vi "AlazarFFTSetScalingAndSlicing.vi"(2 "error in (no error)":errorcluster, 3 "loge_ampl_mult":sgl, 4 "slice_pos":u8, 5 "DSP Handle":u64) -> (0 "error out":errorcluster, 1 "DSP Handle":u64)   [LabVIEW 2018]
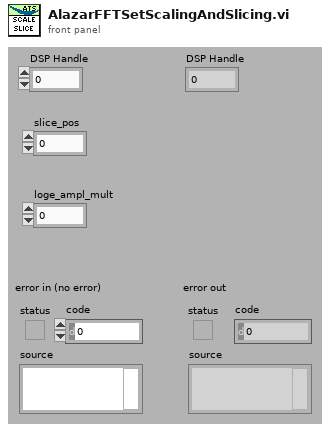
[diagram p1: front panel]
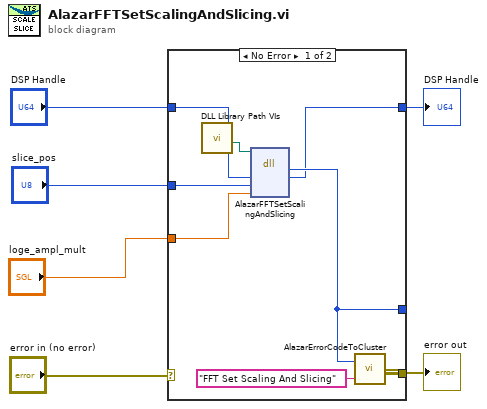
[diagram p0: block diagram]
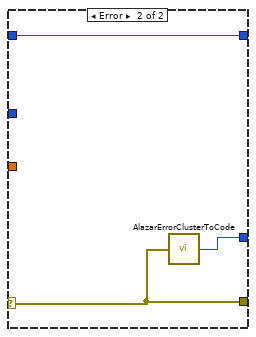
[diagram p2: hidden frame]
diagram:
  n1 = case shown="No Error" "error in (no error)" {
    selector: "error in (no error)" -> [_ w17]
    tunnel: [w11 w17] -> w5
    tunnel: [w13 w16] -> _
    tunnel: "DSP Handle" -> [w14 w15]
    tunnel: [w10 w15] -> w3
    tunnel: "slice_pos" -> [w9 _]
    tunnel: "loge_ampl_mult" -> [w8 _]
    frame No Error {
      n2 = call "DLL Library Path VIs.vi"() -> ("Alazar"=w7:path)  [unwired: 9 in, 2 out]
      n3 = dll-call lib="C:/Project/SerialSectOCT - FFT GPU/SerialSectOCT/Labview Software/DLL/ATSApi.dll" fn="AlazarFFTSetScalingAndSlicing"(path in=w7, "handle"=w14, "slice_pos"=w9, "loge_ampl_mult"=w8) -> ("return type"=w13:u32, "handle"=w10:u64)  [unwired: 4 in, 2 out]
      n4 = call "AlazarErrorCodeToCluster.vi"("Message"="FFT Set Scaling And Slicing", "Error Code"=w13) -> ("error out"=w11:errorcluster)
    }
    frame Error {
      n5 = call "AlazarErrorClusterToCode.vi"("error in (no error)"=w17) -> ("Error Code"=w16:u32)
    }
  }
  "DSP Handle" <- w3
  "error out" <- w5
